vi "Local Mapper C.vi"(11 "GIC Input":T1={"     Use ?\nOff       On"=[FALSE, TRUE, FALSE, TRUE], "Mode:"=FALSE, "WP Data"="", "Hokuyo Port"="COM7", "Prop  Port"="COM6", "Compass Port"="", "GPS Port"="", "Num of WPs"=0, "WP Lats and Longs"={"WP Lats"=[], "WP Longs"=[]}, "Obst Lats and Longs"={"Obst Lats"=[], "Obst Longs"=[]}, "Parameters"=[], "GPS Data"=[], "Compass"=0.0, "LMS Vector"=[], "Vision Vector"=[], "Direction Cmd"=0.0, "Speed Cmd"=0.0, "WP Vector"=[], "WP Number"=0, "Extra"=0, "SW Map"=[], "Path Cluster"={"Path x node"=[], "Path y node"=[]}, "Sim Course"=[]} {"Obst Lats and Longs"."Obst Longs" format="%#_8g"; "Obst Lats and Longs"."Obst Lats" format="%#_8g"}) -> (3 "Local Map":picture)   [LabVIEW 2014]
panel:
  # "Local Mapper C"
  # "Input:"
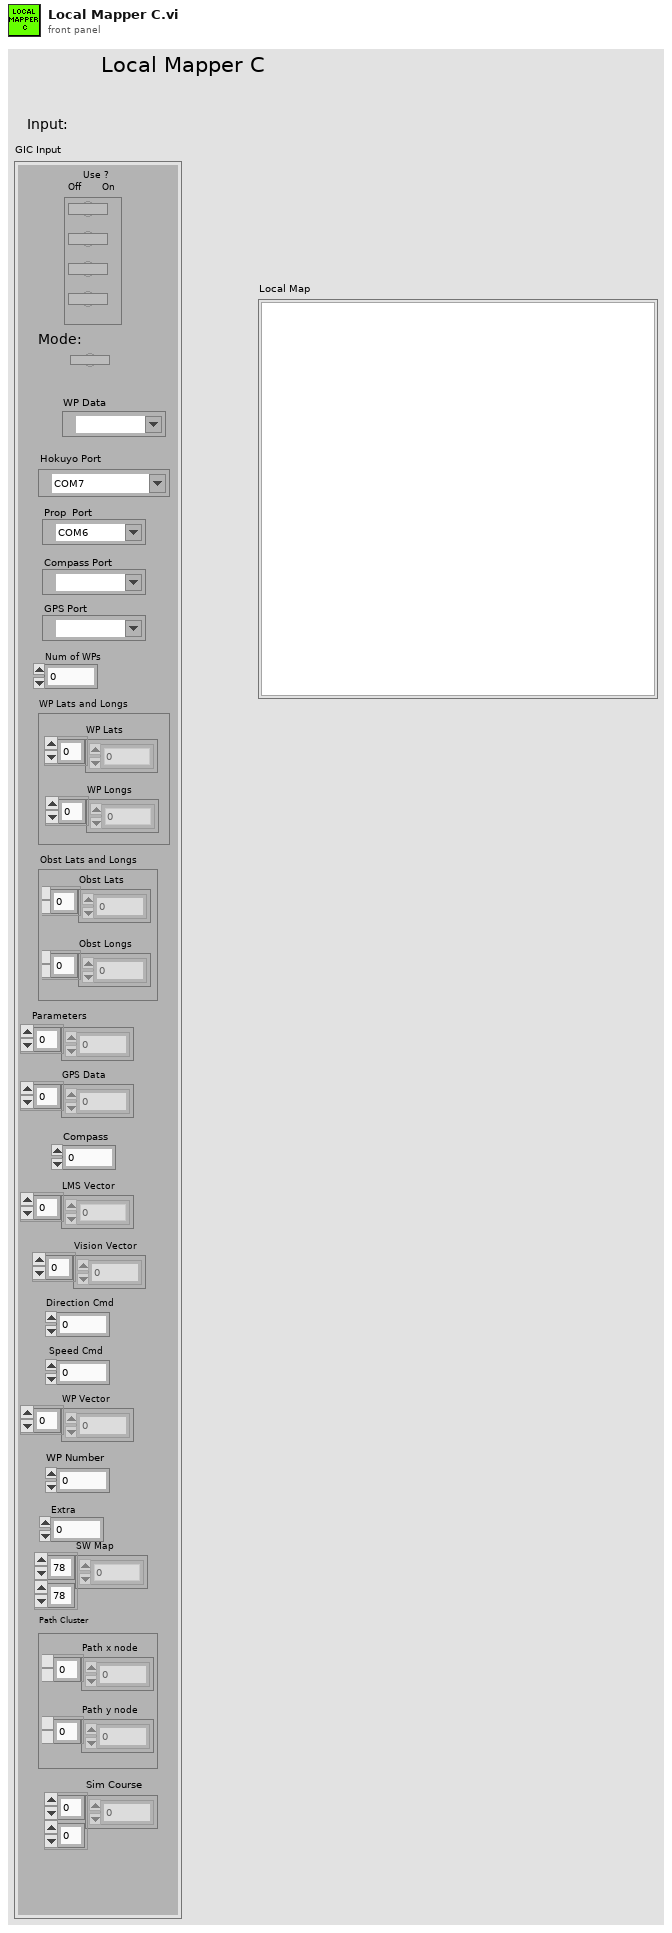
[diagram p1: front panel]
types:
  T1 = cluster{"     Use ?\nOff       On":bool[], "Mode:":bool, "WP Data":refnum<visa-resource-name>, "Hokuyo Port":refnum<visa-resource-name>, "Prop  Port":refnum<visa-resource-name>, "Compass Port":refnum<visa-resource-name>, "GPS Port":refnum<visa-resource-name>, "Num of WPs":i16, "WP Lats and Longs":cluster{"WP Lats":dbl[], "WP Longs":dbl[]}, "Obst Lats and Longs":cluster{"Obst Lats":dbl[], "Obst Longs":dbl[]}, "Parameters":dbl[], "GPS Data":dbl[], "Compass":dbl, "LMS Vector":dbl[], "Vision Vector":dbl[], "Direction Cmd":dbl, "Speed Cmd":dbl, "WP Vector":dbl[], "WP Number":i32, "Extra":i16, "SW Map":i32[][], "Path Cluster":cluster{"Path x node":dbl[], "Path y node":dbl[]}, "Sim Course":i8[][]}
  T2 = cluster{"Width":u16, "Style":enum32{"Solid", "Dash", "Dot", "DashDot", "DashDotDot"}}
  T3 = cluster{"left":i16, "top":i16, "right":i16, "bottom":i16}
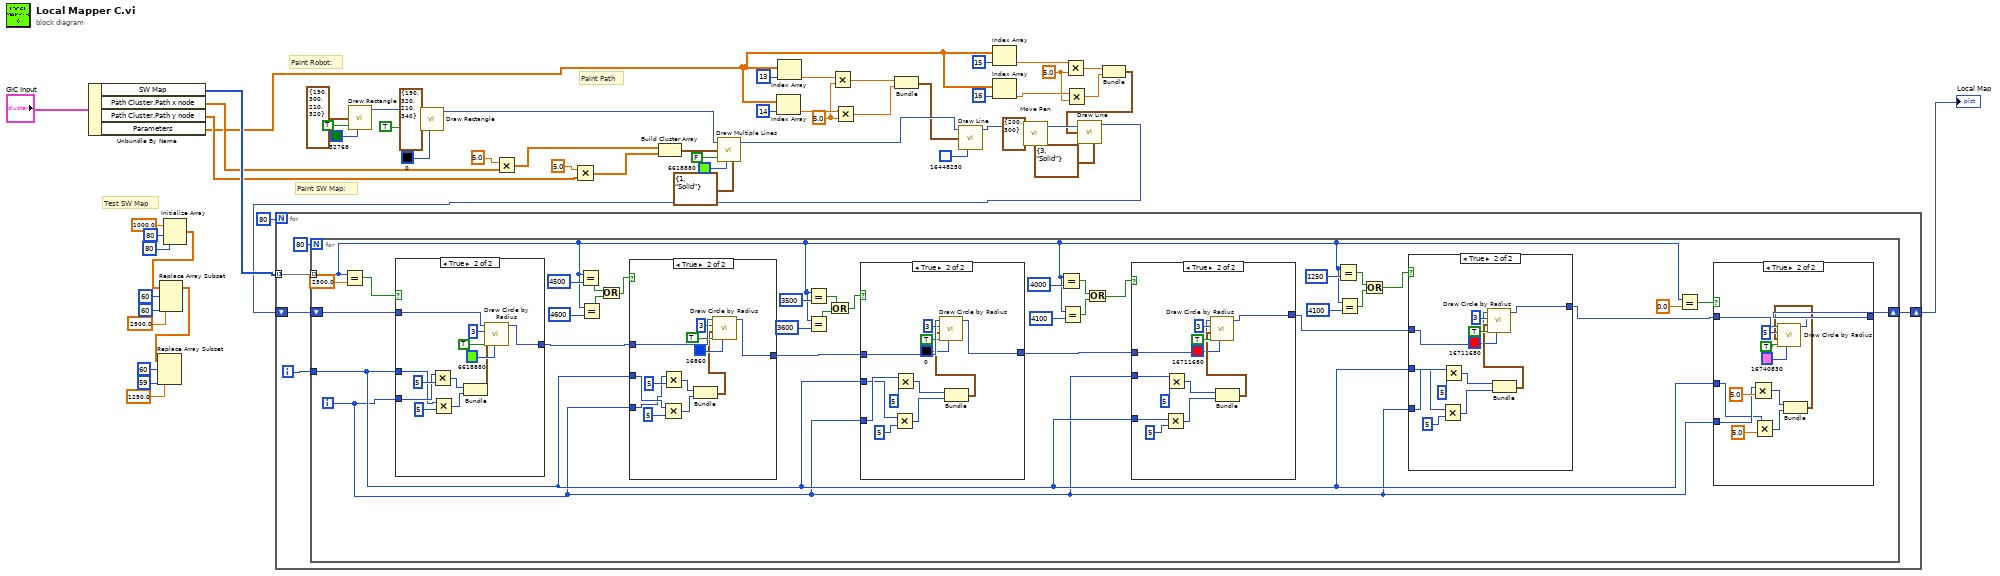
[diagram p0: block diagram]
diagram:
  w5 = 5.0 ("y")
  w18 = 5.0 ("y")
  # "Paint Path"
  # "Test SW Map"
  # "Paint SW Map:"
  # "Paint Robot:"
  n1 = Unbundle By Name("GIC Input") -> ("SW Map"=w37:i32[][], "Path Cluster.Path x node"=w35:dbl[], "Path Cluster.Path y node"=w33:dbl[], "Parameters"=w11:dbl[])
  n2 = Initialize Array(1000.0 ("element"), 80 ("dimension size"), 80 ("dimension size")) -> (w47:dbl[][])
  n3 = Replace Array Subset(array=w47, new element=2500.0 ("new element/subarray"), index (row)=60, index (col)=60 ("disabled index (col)")) -> (w41:dbl[][])
  n4 = Replace Array Subset(array=w41, new element=1250.0 ("new element/subarray"), index (row)=60, index (col)=59 ("disabled index (col)")) -> ()  [unwired: 1 out]
  n5 = call <vilib>:"Draw Rectangle.vi"("rect"=T3 {"left"=190, "top"=300, "right"=210, "bottom"=320}, "fill?(F)"=TRUE, "color(black)"=u32 32768) -> ("new picture"=w54:picture)  [unwired: 6 in]
  n6 = call <vilib>:"Draw Rectangle.vi"("picture"=w54, "rect"=T3 {"left"=190, "top"=320, "right"=210, "bottom"=340}, "fill?(F)"=TRUE, "color(black)"=u32 0) -> ("new picture"=w26:picture)  [unwired: 5 in]
  n7 = Multiply(x=5.0, y=w35) -> (x*y=w32:dbl[])
  n8 = Multiply(x=5.0, y=w33) -> (x*y=w31:dbl[])
  n9 = Build Cluster Array(w32, w31) -> (w30:cluster{dbl, dbl}[])
  n10 = call <vilib>:"Draw Multiple Lines.vi"("picture"=w26, "line endpoints"=w30, "fill?(F)"=FALSE, "color(black)"=u32 6618880, "pen"=T2 {"Width"=1, "Style"=enum."Solid"}) -> ("new picture"=w25:picture)  [unwired: 4 in]
  n11 = Index Array(array=w11, index=14) -> (element=w20:dbl)
  n12 = Index Array(array=w11, index=13) -> (element=w17:dbl)
  n13 = Multiply(x=w17, y=w18) -> (x*y=w16:dbl)
  n14 = Multiply(x=w20, y=w18) -> (x*y=w19:dbl)
  n15 = Bundle(w16, w19) -> (w21:cluster{dbl, dbl})  [unwired: 1 in]
  n16 = call <vilib>:"Draw Line.vi"("picture"=w25, "end point"=w21, "color(black)"=u32 16448250) -> ("new picture"=w13:picture)  [unwired: 6 in]
  n17 = Index Array(array=w11, index=15) -> (element=w7:dbl)
  n18 = Index Array(array=w11, index=16) -> (element=w6:dbl)
  n19 = call <vilib>:"Move Pen.vi"("new position"=cluster{"x":i16, "y":i16} {"x"=200, "y"=300}, "picture"=w13) -> ("new picture"=w14:picture)  [unwired: 3 in]
  n20 = Multiply(x=w7, y=w5) -> (x*y=w8:dbl)
  n21 = Multiply(x=w6, y=w5) -> (x*y=w4:dbl)
  n22 = Bundle(w8, w4) -> (w3:cluster{dbl, dbl})  [unwired: 1 in]
  n23 = call <vilib>:"Draw Line.vi"("picture"=w14, "end point"=w3, "pen"=T2 {"Width"=3, "Style"=enum."Solid"}) -> ("new picture"=w15:picture)  [unwired: 6 in]
  n24 = for {
    N: 80 -> [_]
    tunnel: w37 -> [w61] mode=indexing
    shift-right: [w59] -> w43
    shift-left: w15 -> [w60]
    i -> [w58]
    n25 = for {
      N: 80 -> [_]
      tunnel: w61 -> [w67] mode=indexing
      shift-right: [w91] -> w59
      shift-left: w60 -> [w94]
      tunnel: w58 -> [w65]
      i -> [w64]
      n26 = Equal?(x=w67, y=2500.0) -> (x = y?=w95:bool)
      n27 = case shown="True" w95 {
        tunnel: w94 -> [w162 w171]
        tunnel: [w162 w168] -> w92
        tunnel: w64 -> [_ w164]
        tunnel: w65 -> [_ w163]
        frame False {
        }
        frame True {
          n28 = Multiply(x=w164, y=5) -> (x*y=w167:i32)
          n29 = Multiply(x=w163, y=5) -> (x*y=w166:i32)
          n30 = Bundle(w167, w166) -> (w165:cluster{i32, i32})  [unwired: 1 in]
          n31 = call <vilib>:"Draw Circle by Radius.vi"("color(black)"=u32 6618880, "fill?(F)"=TRUE, "pixel center"=w165, "radius"=i16 3, "picture"=w171) -> ("new picture"=w168:picture)  [unwired: 6 in]
        }
      }
      n32 = Equal?(x=w67, y=4500) -> (x = y?=w83:bool)
      n33 = Equal?(x=w67, y=4600) -> (x = y?=w82:bool)
      n34 = Or(x=w83, y=w82) -> (x .or. y?=w81:bool)
      n35 = case shown="True" w81 {
        tunnel: w92 -> [w149 w161]
        tunnel: [w149 w160] -> w88
        tunnel: w65 -> [_ w151]
        tunnel: w64 -> [_ w150]
        frame False {
        }
        frame True {
          n36 = Multiply(x=w151, y=5) -> (x*y=w153:i32)
          n37 = Multiply(x=w150, y=5) -> (x*y=w154:i32)
          n38 = Bundle(w154, w153) -> (w152:cluster{i32, i32})  [unwired: 1 in]
          n39 = call <vilib>:"Draw Circle by Radius.vi"("color(black)"=u32 16860, "fill?(F)"=TRUE, "pixel center"=w152, "radius"=i16 3, "picture"=w161) -> ("new picture"=w160:picture)  [unwired: 6 in]
        }
      }
      n40 = Equal?(x=w67, y=3500) -> (x = y?=w75:bool)
      n41 = Equal?(x=w67, y=3600) -> (x = y?=w74:bool)
      n42 = Or(x=w75, y=w74) -> (x .or. y?=w73:bool)
      n43 = case shown="True" w73 {
        tunnel: w88 -> [w123 w135]
        tunnel: [w123 w125] -> w85
        tunnel: w65 -> [_ w129]
        tunnel: w64 -> [_ w130]
        frame False {
        }
        frame True {
          n44 = Multiply(x=w129, y=5) -> (x*y=w132:i32)
          n45 = Multiply(x=w130, y=5) -> (x*y=w131:i32)
          n46 = Bundle(w131, w132) -> (w126:cluster{i32, i32})  [unwired: 1 in]
          n47 = call <vilib>:"Draw Circle by Radius.vi"("color(black)"=u32 0, "fill?(F)"=TRUE, "pixel center"=w126, "radius"=i16 3, "picture"=w135) -> ("new picture"=w125:picture)  [unwired: 6 in]
        }
      }
      n48 = Equal?(x=w67, y=4000) -> (x = y?=w79:bool)
      n49 = Equal?(x=w67, y=4100) -> (x = y?=w78:bool)
      n50 = Or(x=w79, y=w78) -> (x .or. y?=w77:bool)
      n51 = case shown="True" w77 {
        tunnel: [w110 w115] -> w66
        tunnel: w85 -> [w110 w113]
        tunnel: w65 -> [_ w111]
        tunnel: w64 -> [_ w112]
        frame False {
        }
        frame True {
          n52 = Multiply(x=w111, y=5) -> (x*y=w120:i32)
          n53 = Multiply(x=w112, y=5) -> (x*y=w119:i32)
          n54 = Bundle(w119, w120) -> (w116:cluster{i32, i32})  [unwired: 1 in]
          n55 = call <vilib>:"Draw Circle by Radius.vi"("color(black)"=u32 16711680, "fill?(F)"=TRUE, "pixel center"=w116, "radius"=i16 3, "picture"=w113) -> ("new picture"=w115:picture)  [unwired: 6 in]
        }
      }
      n56 = Equal?(x=w67, y=1250) -> (x = y?=w70:bool)
      n57 = Equal?(x=w67, y=4100) -> (x = y?=w71:bool)
      n58 = Or(x=w70, y=w71) -> (x .or. y?=w72:bool)
      n59 = case shown="True" w72 {
        tunnel: [w97 w102] -> w63
        tunnel: w66 -> [w97 w100]
        tunnel: w65 -> [_ w98]
        tunnel: w64 -> [_ w99]
        frame False {
        }
        frame True {
          n60 = Multiply(x=w98, y=5) -> (x*y=w107:i32)
          n61 = Multiply(x=w99, y=5) -> (x*y=w106:i32)
          n62 = Bundle(w106, w107) -> (w103:cluster{i32, i32})  [unwired: 1 in]
          n63 = call <vilib>:"Draw Circle by Radius.vi"("color(black)"=u32 16711680, "fill?(F)"=TRUE, "pixel center"=w103, "radius"=i16 3, "picture"=w100) -> ("new picture"=w102:picture)  [unwired: 6 in]
        }
      }
      n64 = Equal?(x=w67, y=0.0) -> (x = y?=w90:bool)
      n65 = case shown="True" w90 {
        tunnel: w63 -> [w136 w148]
        tunnel: [w136 w147] -> w91
        tunnel: w65 -> [_ w138]
        tunnel: w64 -> [_ w139]
        frame False {
        }
        frame True {
          n66 = Multiply(x=w139, y=5.0) -> (x*y=w142:i32)
          n67 = Multiply(x=w138, y=5.0) -> (x*y=w141:i32)
          n68 = Bundle(w142, w141) -> (w140:cluster{i32, i32})  [unwired: 1 in]
          n69 = call <vilib>:"Draw Circle by Radius.vi"("color(black)"=u32 16740830, "fill?(F)"=TRUE, "pixel center"=w140, "radius"=i16 5, "picture"=w148) -> ("new picture"=w147:picture)  [unwired: 6 in]
        }
      }
    }
  }
  "Local Map" <- w43
